vi "Camera Process.vi"(0 "error in":errorcluster) -> ()   [LabVIEW 2012]
uses:
  Camera Global Data.vi
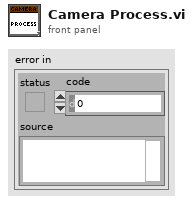
[diagram p1: front panel]
types:
  T1 = cluster{"Y Axis":dbl, "X Axis":dbl, "View Ground":bool, "Center On Target":bool, "Stop Auto move?":bool, "Servo X Current":dbl, "Servo Y Current":dbl, "Target Info":cluster{"Target Found?":bool, "Target X Position":dbl, "Target Y Position":dbl}, "Seen Floor X Angle":dbl, "Seen Floor Y Angle":dbl, "Centerd?":bool, "Servo X Set":dbl, "Servo Y Set":dbl}
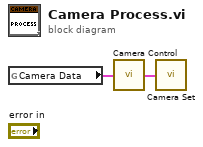
[diagram p0: block diagram]
diagram:
  n1 = global read "Camera Global Data.vi" "Camera Data"() -> (w1:T1)
  n2 = call "Camera Control.vi"("Camera Data"=w1) -> ("Camera Data out"=w2:T1)
  n3 = call "Camera Set.vi"("Camera Data"=w2) -> ()
